vi "write channel state.vi"(8 "error in (no error)":errorcluster, 10 "State":string, 11 "S4GEI in":refnum<class "S4GEI.lvclass">) -> (0 "error out":errorcluster, 3 "S4GEI out":refnum<class "S4GEI.lvclass">)   [LabVIEW 2018, in "S4GEI.lvclass"]
uses:
  S4GEI.lvclass
  S4GEI.lvclass/S4GEI.ctl
  Channel GUI/Channel.lvclass
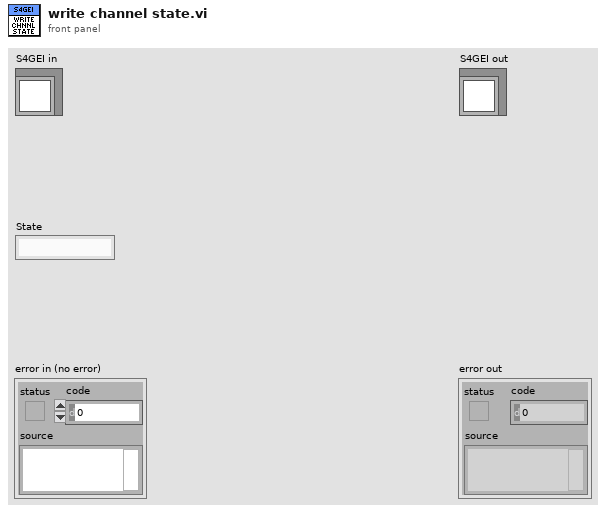
[diagram p1: front panel]
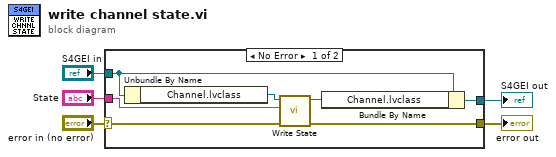
[diagram p0: block diagram]
diagram:
  n1 = case shown="No Error" "error in (no error)" {
    selector: "error in (no error)" -> [w8 w14]
    tunnel: [w7 w14] -> w4
    tunnel: [w11 w13] -> w2
    tunnel: "S4GEI in" -> [w12 w13]
    tunnel: "State" -> [w6 _]
    frame No Error {
      n2 = Unbundle By Name(w12) -> ("Channel.lvclass"=w10:refnum<class "Channel.lvclass">)
      n3 = call "Write State.vi"("error in (no error)"=w8, "State"=w6, "Channel GEI in"=w10) -> ("error out"=w7:errorcluster, "Channel GEI out"=w9:refnum<class "Channel.lvclass">)  [unwired: 7 in]
      n4 = Bundle By Name(cluster=w12, "Channel.lvclass"=w9) -> (w11:refnum<class "S4GEI.lvclass">)
    }
    frame Error {
    }
  }
  "error out" <- w4
  "S4GEI out" <- w2
